vi "Test FindLogItemsInJson.vi"(8 "error in (no error)":errorcluster) -> (0 "error out":errorcluster)   [LabVIEW 2017, in "UT_LokiJsonFormatter.lvlib"]
doc: "Template for an unit test with caraya in the \"Given, When, Then\" structure from James."
uses:
  UT_LokiJsonFormatter.lvlib
  <vilib>/addons/_JKI Toolkits/Caraya/classes/Test/Test.lvclass
  <vilib>/addons/_JKI Toolkits/Caraya/classes/Assert/Assert.lvclass
  Source/HSE-Logger/Formatter/LokiJsonFormatter/LokiJsonFormatter.lvclass
  Source/HSE-Logger/LogRecord/LogRecord.lvclass
  Source/HSE-Logger/LogLevel.ctl
  Source/HSE-Logger/hse-logger.lvlib
  <vilib>/addons/_JKI Toolkits/Caraya/classes/Assert/Assert True.vi
panel:
  # "Connector Pane"
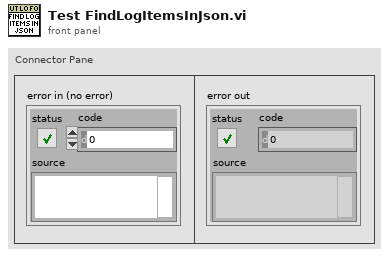
[diagram p1: front panel]
types:
  T1 = typedef "hse-logger.lvlib/LogLevel.ctl" = enum16{"DEBUG", "INFO", "WARNING", "ERROR", "CRITICAL"}
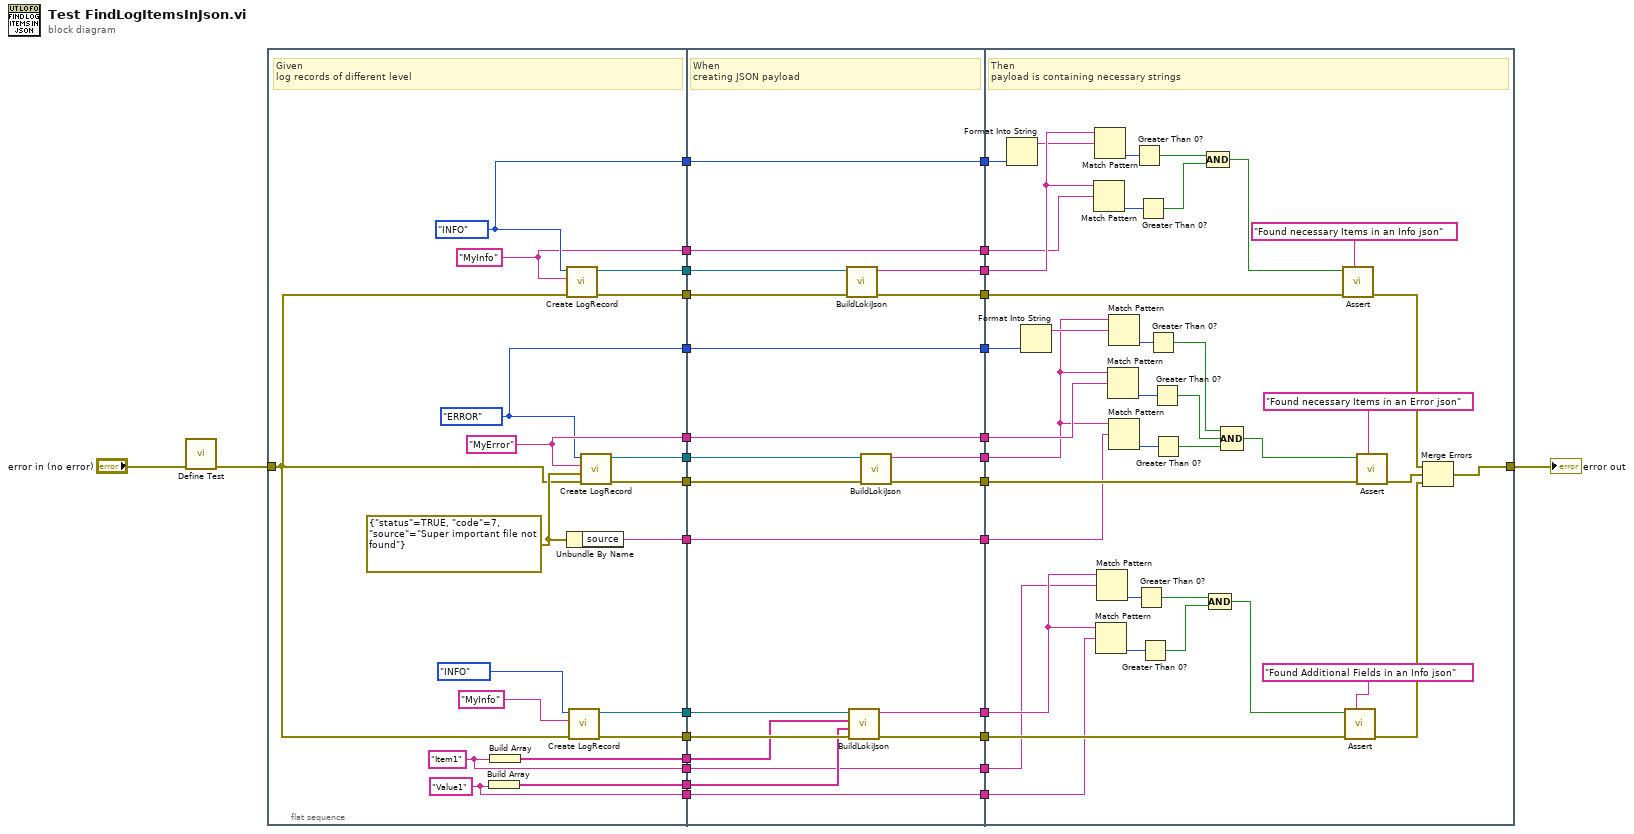
[diagram p0: block diagram]
diagram:
  n1 = call <vilib>:"Define Test.vi"("error in (no error)"="error in (no error)") -> ("error out"=w28:errorcluster)  [unwired: 9 in, 1 out]
  n2 = flat-sequence {
    tunnel: w28 -> [w36]
    tunnel: [w47] -> w31
    tunnel: [w50] -> w25
    tunnel: [w49] -> w24
    tunnel: [w48] -> w21
    tunnel: [w46] -> w16
    tunnel: [w43] -> w15
    tunnel: [w44] -> w14
    tunnel: [w45] -> w13
    tunnel: [w41] -> w12
    tunnel: [w40] -> w8
    tunnel: [w37] -> w7
    tunnel: [w35] -> w6
    tunnel: [w34] -> w5
    tunnel: [w33] -> w4
    tunnel: [w32] -> w2
    tunnel: w31 -> [w70]
    tunnel: [w71] -> w27
    tunnel: [w69] -> w26
    tunnel: w25 -> [w68]
    tunnel: w24 -> [w67]
    tunnel: [w67] -> w23
    tunnel: [w66] -> w22
    tunnel: w21 -> [w66]
    tunnel: [w60] -> w20
    tunnel: [w62] -> w19
    tunnel: [w64] -> w18
    tunnel: [w65] -> w17
    tunnel: w16 -> [w61]
    tunnel: w15 -> [w63]
    tunnel: w14 -> [w64]
    tunnel: w13 -> [w65]
    tunnel: w12 -> [w59]
    tunnel: [w59] -> w11
    tunnel: [w55] -> w10
    tunnel: [w57] -> w9
    tunnel: w8 -> [w56]
    tunnel: w7 -> [w58]
    tunnel: w6 -> [w54]
    tunnel: w5 -> [w53]
    tunnel: w4 -> [w52]
    tunnel: [w52] -> w3
    tunnel: w2 -> [w51]
    tunnel: [w51] -> w1
    tunnel: [w109] -> w30
    tunnel: w27 -> [w107]
    tunnel: w26 -> [w106]
    tunnel: w23 -> [w104]
    tunnel: w22 -> [w103]
    tunnel: w20 -> [w89]
    tunnel: w19 -> [w84]
    tunnel: w18 -> [w91]
    tunnel: w17 -> [w92]
    tunnel: w11 -> [w83]
    tunnel: w10 -> [w76]
    tunnel: w9 -> [w77]
    tunnel: w3 -> [w73]
    tunnel: w1 -> [w72]
    frame #0 {
      w32 = "Value1" ("Name")
      w33 = "Item1" ("Name")
      w42 = errorcluster {"status"=TRUE, "code"=7, "source"="Super important file not found"} ("Error to Log")
      w45 = "MyError" ("Message")
      w44 = LogLevel."ERROR" ("Level")
      w48 = "MyInfo" ("Message")
      w49 = LogLevel."INFO" ("Level")
      # "Given\nlog records of different level"
      n3 = Build Array(w32) -> (w34:string[])
      n4 = Build Array(w33) -> (w35:string[])
      n5 = call "Create LogRecord.vi"("error in"=w36, "Message"=w48, "Level"=w49) -> ("error out"=w47:errorcluster, "LogRecord out"=w50:refnum<class "LogRecord.lvclass">)  [unwired: 7 in]
      n6 = Unbundle By Name(w42) -> ("source"=w41:string)
      n7 = call "Create LogRecord.vi"("error in"=w36, "Message"="MyInfo", "Level"=LogLevel."INFO") -> ("error out"=w40:errorcluster, "LogRecord out"=w37:refnum<class "LogRecord.lvclass">)  [unwired: 7 in]
      n8 = call "Create LogRecord.vi"("error in"=w36, "Error to Log"=w42, "Message"=w45, "Level"=w44) -> ("error out"=w46:errorcluster, "LogRecord out"=w43:refnum<class "LogRecord.lvclass">)  [unwired: 6 in]
    }
    frame #1 {
      # "When\ncreating JSON payload"
      n9 = call "BuildLokiJson.vi"("error in (no error)"=w70, "LogRecord"=w68) -> ("error out"=w71:errorcluster, "<JSON> out"=w69:string)  [unwired: 8 in]
      n10 = call "BuildLokiJson.vi"("error in (no error)"=w56, "Stream Fields Values"=w53, "Stream Fields"=w54, "LogRecord"=w58) -> ("error out"=w55:errorcluster, "<JSON> out"=w57:string)  [unwired: 6 in]
      n11 = call "BuildLokiJson.vi"("error in (no error)"=w61, "LogRecord"=w63) -> ("error out"=w60:errorcluster, "<JSON> out"=w62:string)  [unwired: 8 in]
    }
    frame #2 {
      # "Then\npayload is containing necessary strings"
      n12 = Format Into String(w104) -> (resulting string=w105:string)  [unwired: 3 in, 1 out]
      n13 = Format Into String(w91) -> (resulting string=w90:string)  [unwired: 3 in, 1 out]
      n14 = Match Pattern(string=w106, regular expression=w103) -> (offset past match=w101:i32)  [unwired: 1 in, 3 out]
      n15 = Match Pattern(string=w106, regular expression=w105) -> (offset past match=w102:i32)  [unwired: 1 in, 3 out]
      n16 = Match Pattern(string=w77, regular expression=w72) -> (offset past match=w79:i32)  [unwired: 1 in, 3 out]
      n17 = Match Pattern(string=w77, regular expression=w73) -> (offset past match=w78:i32)  [unwired: 1 in, 3 out]
      n18 = Match Pattern(string=w84, regular expression=w92) -> (offset past match=w94:i32)  [unwired: 1 in, 3 out]
      n19 = Match Pattern(string=w84, regular expression=w90) -> (offset past match=w93:i32)  [unwired: 1 in, 3 out]
      n20 = Match Pattern(string=w84, regular expression=w83) -> (offset past match=w86:i32)  [unwired: 1 in, 3 out]
      n21 = Greater Than 0?(x=w102) -> (x > 0?=w100:bool)
      n22 = Greater Than 0?(x=w78) -> (x > 0?=w80:bool)
      n23 = Greater Than 0?(x=w101) -> (x > 0?=w99:bool)
      n24 = Greater Than 0?(x=w79) -> (x > 0?=w81:bool)
      n25 = Greater Than 0?(x=w93) -> (x > 0?=w95:bool)
      n26 = Greater Than 0?(x=w94) -> (x > 0?=w96:bool)
      n27 = Greater Than 0?(x=w86) -> (x > 0?=w85:bool)
      n28 = Compound Arithmetic op=AND(w100, w99) -> (w98:bool)
      n29 = Compound Arithmetic op=AND(w80, w81) -> (w82:bool)
      n30 = Compound Arithmetic op=AND(w95, w96, w85) -> (w97:bool)
      n31 = call-poly <vilib>:"Assert.vi"("Label"="Found necessary Items in an Info json", "error in (no error)"=w107, "True?"=w98) -> ("error out"=w110:errorcluster)  [unwired: 7 in, 1 out]
      n32 = call-poly <vilib>:"Assert.vi"("Label"="Found Additional Fields in an Info json", "error in (no error)"=w76, "True?"=w82) -> ("error out"=w74:errorcluster)  [unwired: 7 in, 1 out]
      n33 = call-poly <vilib>:"Assert.vi"("Label"="Found necessary Items in an Error json", "error in (no error)"=w89, "True?"=w97) -> ("error out"=w87:errorcluster)  [unwired: 7 in, 1 out]
      n34 = Merge Errors(w110, w87, w74) -> (w109:errorcluster)
    }
  }
  "error out" <- w30
